vi "Unregister and Destroy User Event.vi"(8 "error in":errorcluster, 11 "UserEventMessageTransport":refnum<class "UserEventMessageTransport.lvclass">) -> (0 "error out":errorcluster, 3 "UserEventMessageTransport":refnum<class "UserEventMessageTransport.lvclass">)   [LabVIEW 2016, in "UserEventMessageTransport.lvclass"]
uses:
  UserEventMessageTransport.lvclass
  UserEventMessageTransport.lvclass/UserEventMessageTransport.ctl
  IMessagePayload/IMessagePayload.lvclass
panel:
  # "INPUTS"
  # "OUTPUTS"
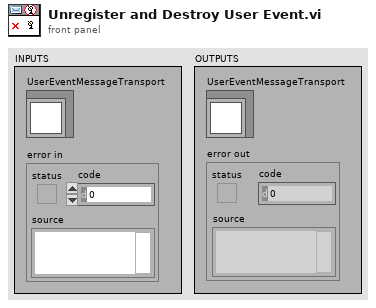
[diagram p1: front panel]
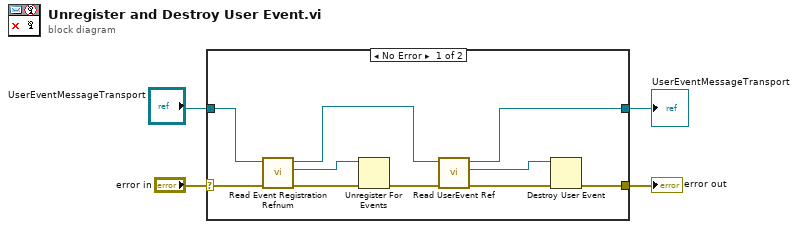
[diagram p0: block diagram]
diagram:
  n1 = case shown="No Error" "error in" {
    selector: "error in" -> [w6 w15]
    tunnel: [w9 w16] -> w2
    tunnel: "UserEventMessageTransport" -> [w14 w16]
    tunnel: [w5 w15] -> w1
    frame No Error {
      n2 = call "Read Event Registration Refnum.vi"("error in"=w6, "UserEventMessageTransport in"=w14) -> ("error out"=w13:errorcluster, "Event Registration Refnum"=w12:refnum<event-registration>, "UserEventMessageTransport out"=w10:refnum<class "UserEventMessageTransport.lvclass">)  [unwired: 7 in]
      n3 = Unregister For Events(event registration refnum=w12, error in=w13) -> (error out=w11:errorcluster)
      n4 = call "Read UserEvent Ref.vi"("error in"=w11, "UserEventMessageTransport in"=w10) -> ("error out"=w8:errorcluster, "UserEvent Ref"=w7:refnum<user-event>, "UserEventMessageTransport out"=w9:refnum<class "UserEventMessageTransport.lvclass">)  [unwired: 7 in]
      n5 = Destroy User Event(user event=w7, error in=w8) -> (error out=w5:errorcluster)
    }
    frame Error {
    }
  }
  "error out" <- w1
  "UserEventMessageTransport" <- w2
